vi "Open Sensors and Actuators.vi"   [LabVIEW 2014]
uses:
  <vilib>/Rock Robotics/SystemInterfaces/DIO/FPGA_DIOPWMChannel.ctl
  <vilib>/Rock Robotics/WPI/Joystick/WPI_JoystickDeviceEnum.ctl
  <vilib>/Rock Robotics/SystemInterfaces/DIO/FPGA_DIOChannel.ctl
  <vilib>/Rock Robotics/WPI/Solenoid/WPI_SolenoidChannel.ctl
  <vilib>/Rock Robotics/SystemInterfaces/AI/FPGA_AIChannel.ctl
  <vilib>/Rock Robotics/WPI/MotorControl/WPI_MotorControlOpen Talon.vi
  <vilib>/Rock Robotics/WPI/Counter/WPI_CounterDigitalInputToDigitalSource.vi
  <vilib>/Rock Robotics/WPI/Solenoid/WPI_SolenoidOpenSingle.vi
  <vilib>/Rock Robotics/WPI/Counter/WPI_CounterOpen UpDown Mode.vi
  <vilib>/Rock Robotics/WPI/Switch/WPI_SwitchOpenLimit.vi
  <vilib>/Rock Robotics/WPI/Ultrasonic/WPI_SonarMB1010AnalogOpen.vi
  Global RefNums.vi
  <vilib>/Rock Robotics/WPI/Compressor/WPI_CompressorGetSetRefNum.vi
  <vilib>/Rock Robotics/WPI/Ultrasonic/WPI_SonarMB1010AnalogRefNum Registry Set.vi
  _Dependencies/NavX/navX-MXP IMU.lvlib
types:
  T1 = typedef "WPI_SolenoidChannel.ctl" = enum8{"Solenoid 0", "Solenoid 1", "Solenoid 2", "Solenoid 3", "Solenoid 4", "Solenoid 5", "Solenoid 6", "Solenoid 7", "Invalid"}
  T2 = typedef "FPGA_AIChannel.ctl" = enum8{"AI 0", "AI 1", "AI 2", "AI 3", "AI MXP 0", "AI MXP 1", "AI MXP 2", "AI MXP 3", "Invalid"}
  T3 = typedef "FPGA_DIOChannel.ctl" = enum8{"DIO 0", "DIO 1", "DIO 2", "DIO 3", "DIO 4", "DIO 5", "DIO 6", "DIO 7", "DIO 8", "DIO 9", "DIO MXP 0", "DIO MXP 1", "DIO MXP 2", "DIO MXP 3", "DIO MXP 4", "DIO MXP 5", "DIO MXP 6", "DIO MXP 7", "DIO MXP 8", "DIO MXP 9", "DIO MXP 10", "DIO MXP 11", "DIO MXP 12", "DIO MXP 13", "DIO MXP 14", "DIO MXP 15", "Invalid"}
  T4 = typedef "FPGA_DIOPWMChannel.ctl" = enum8{"PWM 0", "PWM 1", "PWM 2", "PWM 3", "PWM 4", "PWM 5", "PWM 6", "PWM 7", "PWM 8", "PWM 9", "PWM MXP 0", "PWM MXP 1", "PWM MXP 2", "PWM MXP 3", "PWM MXP 4", "PWM MXP 5", "PWM MXP 6", "PWM MXP 7", "PWM MXP 8", "PWM MXP 9", "Invalid"}
  T5 = enum16{"Rising Edge", "Falling Edge", "Raising & Falling Edge", "Disabled"}
  T6 = typedef "WPI_JoystickDeviceEnum.ctl" = enum16{"USB 0", "USB 1", "USB 2", "USB 3", "USB 4", "USB 5"}
  T7 = typedef "WPI_MotorControlDeviceRef.ctl" = cluster{"DeviceStatus":errorcluster, "Type":T8, "PWM":cluster{"Controller":T9, "PWM Channel":T4, "DeadBand":T10}, "CAN":cluster{"Device Number":u8, "Control Mode":T11, "Semaphore":T12, "Max Vout":dbl, "TalonSRX Control Mode":T13}, "Invert":bool, "TransformRef":T14, "InvTransformRef":T14}
  T8 = typedef "WPI_MotorControlType.ctl" = enum16{"PWM", "CAN", "CANTalonSRX"}
  T9 = typedef "FPGA_TypedefDigitalModule.ctl" = enum16{"Controller 1"}
  T10 = typedef "WPI_PWMDeadband.ctl" = cluster{"Name":string, "maxPositivePwm":i32, "minPositivePwm":i32, "centerPwm":i32, "maxNegativePwm":i32, "minNegativePwm":i32, "angularRange":u16}
  T11 = typedef "WPI_CANJaguar_ControlMode.ctl" = enum8{"Percent VBus", "Current", "Speed", "Position", "Voltage"}
  T12 = typedef "Semaphore RefNum" = refnum<k1>
  T13 = typedef "WPI_CANTalonSRX_APIControlMode.ctl" = enum8{"Percent VBus", "Speed", "Position", "Slave", "Unchanged / Invalid"}
  T14 = typedef "WPI_PWMTransform_ConPane.ctl" = refnum<vi>
  T15 = typedef "WPI_DigitalInputDevRef.ctl" = cluster{"DevStatus":errorcluster, "DIO Channel":T3, "Controller":T9}
  T16 = typedef "FPGA_CounterEncoderSourceConvertionLVSourceType.ctl" = cluster{"DevStatus":errorcluster, "AnalogTriggerMode?":bool, "DigitalMode":cluster{"Controller":T9, "DIO Channel":T17}, "AnalogTriggerMode":cluster{"AnalogTriggerIndex":T18, "OutputType":T19}}
  T17 = typedef "FPGA_DIODigitalSourceChannel.ctl" = enum8{"DIO 0", "DIO 1", "DIO 2", "DIO 3", "DIO 4", "DIO 5", "DIO 6", "DIO 7", "DIO 8", "DIO 9", "DIO MXP 0", "DIO MXP 1", "DIO MXP 2", "DIO MXP 3", "DIO MXP 4", "DIO MXP 5", "DIO MXP 6", "DIO MXP 7", "DIO MXP 8", "DIO MXP 9", "DIO MXP 10", "DIO MXP 11", "DIO MXP 12", "DIO MXP 13", "DIO MXP 14", "DIO MXP 15", "Disabled"}
  T18 = typedef "FPGA_AnalogTriggerIndex.ctl" = enum8{"Trig 0", "Trig 1", "Trig 2", "Trig 3", "Trig 4", "Trig 5", "Trig 6", "Trig 7", "Invalid"}
  T19 = typedef "FPGA_AnalogTriggerOutType.ctl" = enum16{"InWindow", "TriggerState", "Rising", "Falling"}
  T20 = typedef "WPI_EncoderDevRef.ctl" = cluster{"DevStatus":errorcluster, "EncoderIndex":T21, "CounterIndex":T22, "DistancePerCount":dbl, "Decoding Type":T23}
  T21 = typedef "FPGA_EncoderIdx.ctl" = enum8{"Enc 0", "Enc 1", "Enc 2", "Enc 3", "Enc 4", "Enc 5", "Enc 6", "Enc 7", "Invalid"}
  T22 = typedef "FPGA_CounterCtrSystemIndex.ctl" = enum8{"Ctr 0", "Ctr 1", "Ctr 2", "Ctr 3", "Ctr 4", "Ctr 5", "Ctr 6", "Ctr 7", "Invalid"}
  T23 = typedef "WPI_EncoderType.ctl" = enum16{"1x", "2x", "4x"}
  T24 = typedef "navX-MXP IMU.lvlib/navX Device TypeDef.ctl" = cluster{"navX Interface Protocol":T25, "navX Interface Protocol TypeDefs":cluster{"SPIDevRef":T26, "I2CDevRef":T28}, "navX System Information":cluster{"Board Information":T30, "Status":T31, "Offsets":T35}, "navX Common Information":cluster{"Update Rate (4Hz-60Hz)":T36, "refnum name":string, "error":errorcluster}}
  T25 = typedef "navX-MXP IMU.lvlib/navX Interface Protocol.ctl" = enum16{"SPI", "I2C"}
  T26 = typedef "WPI_SPIDevRef.ctl" = cluster{"DevStatus":errorcluster, "Handle":i32, "Controller":T9, "SPI Bus":T27}
  T27 = typedef "spi_bus.ctl" = enum16{"SPI On-Board, CS0", "SPI On-Board, CS1", "SPI On-Board, CS2", "SPI On-Board, CS3", "SPI MXP", "Invalid"}
  T28 = typedef "WPI_I2CDevRef.ctl" = cluster{"DevStatus":errorcluster, "Controller":T9, "Device Address":u8, "Handle":i32, "I2C Bus":T29}
  T29 = typedef "i2c_bus.ctl" = enum16{"I2C On-Board", "I2C MXP", "Invalid"}
  T30 = typedef "navX-MXP IMU.lvlib/navX Board Information.ctl" = cluster{"WhoAmI (50 | 0x32)":u8, "Board Revision":u8, "Firmware Major Version":u8, "Firmware Minor Version":u8}
  T31 = typedef "navX-MXP IMU.lvlib/navX Status Data.ctl" = cluster{"Update Rate Hz":u8, "Accelerometer Full-Scale Range":u8, "Gyro Full-Scale Range":u16, "NAVX_OP_STATUS":T32, "NAVX_CAL_STATUS":T33, "NAVX_SELFTEST_STATUS":u8, "NAVX_SENSOR_STATUS":T34}
  T32 = typedef "navX-MXP IMU.lvlib/navX NAVX_OP_STATUS.ctl" = u8
  T33 = typedef "navX-MXP IMU.lvlib/navX NAVX_CAL_STATUS.ctl" = u8
  T34 = typedef "navX-MXP IMU.lvlib/navX NAVX_SENSOR_STATUS.ctl" = cluster{"MOVING":bool, "YAW_STABLE":bool, "MAG_DISTURBANCE":bool, "ALTITUDE_VALID":bool, "SEALEVEL_PRESS_SET":bool, "FUSED_HEADING_VALID":bool}
  T35 = typedef "navX-MXP IMU.lvlib/navX Offsets Data.ctl" = cluster{"Yaw":dbl, "Quat W":dbl, "Quat X":dbl, "Quat Y":dbl, "Quat Z":dbl}
  T36 = typedef "navX-MXP IMU.lvlib/navX Update Rate.ctl" = u8
  T37 = typedef "WPI_JoystickDevRef.ctl" = cluster{"Device":T6}
  T38 = typedef "WPI_SolenoidDevRef.ctl" = cluster{"DevStatus":errorcluster, "Pneumatics Control Module":u8, "Forward Solenoid Channel":T1, "Reverse Solenoid Channel":T1}
  T39 = typedef "WPI_AnalogChannelDevRef.ctl" = cluster{"DevStatus":errorcluster, "Controller":T40, "Analog Channel":T2}
  T40 = typedef "FPGA_TypedefAnalogModule.ctl" = enum16{"Controller 1"}
  T41 = typedef "WPI_CounterDevRef.ctl" = cluster{"DevStatus":errorcluster, "CntIndex":T22}
  T42 = typedef "WPI_CompressorDevRef.ctl" = cluster{"DevStatus":errorcluster, "Pneumatics Control Module":u8}
  T43 = typedef "WPI_SwitchDevRef.ctl" = cluster{"DevStatus":errorcluster, "DIO Channel":T3, "Controller":T9, "CntIndex":T22, "Normally Closed":bool}
  T44 = typedef "WPI_SonarMB1010AnalogDeviceRef.ctl" = cluster{"AIDeviceRef":T39, "Scaling factor (V/in)":dbl, "Average Bits":u8}
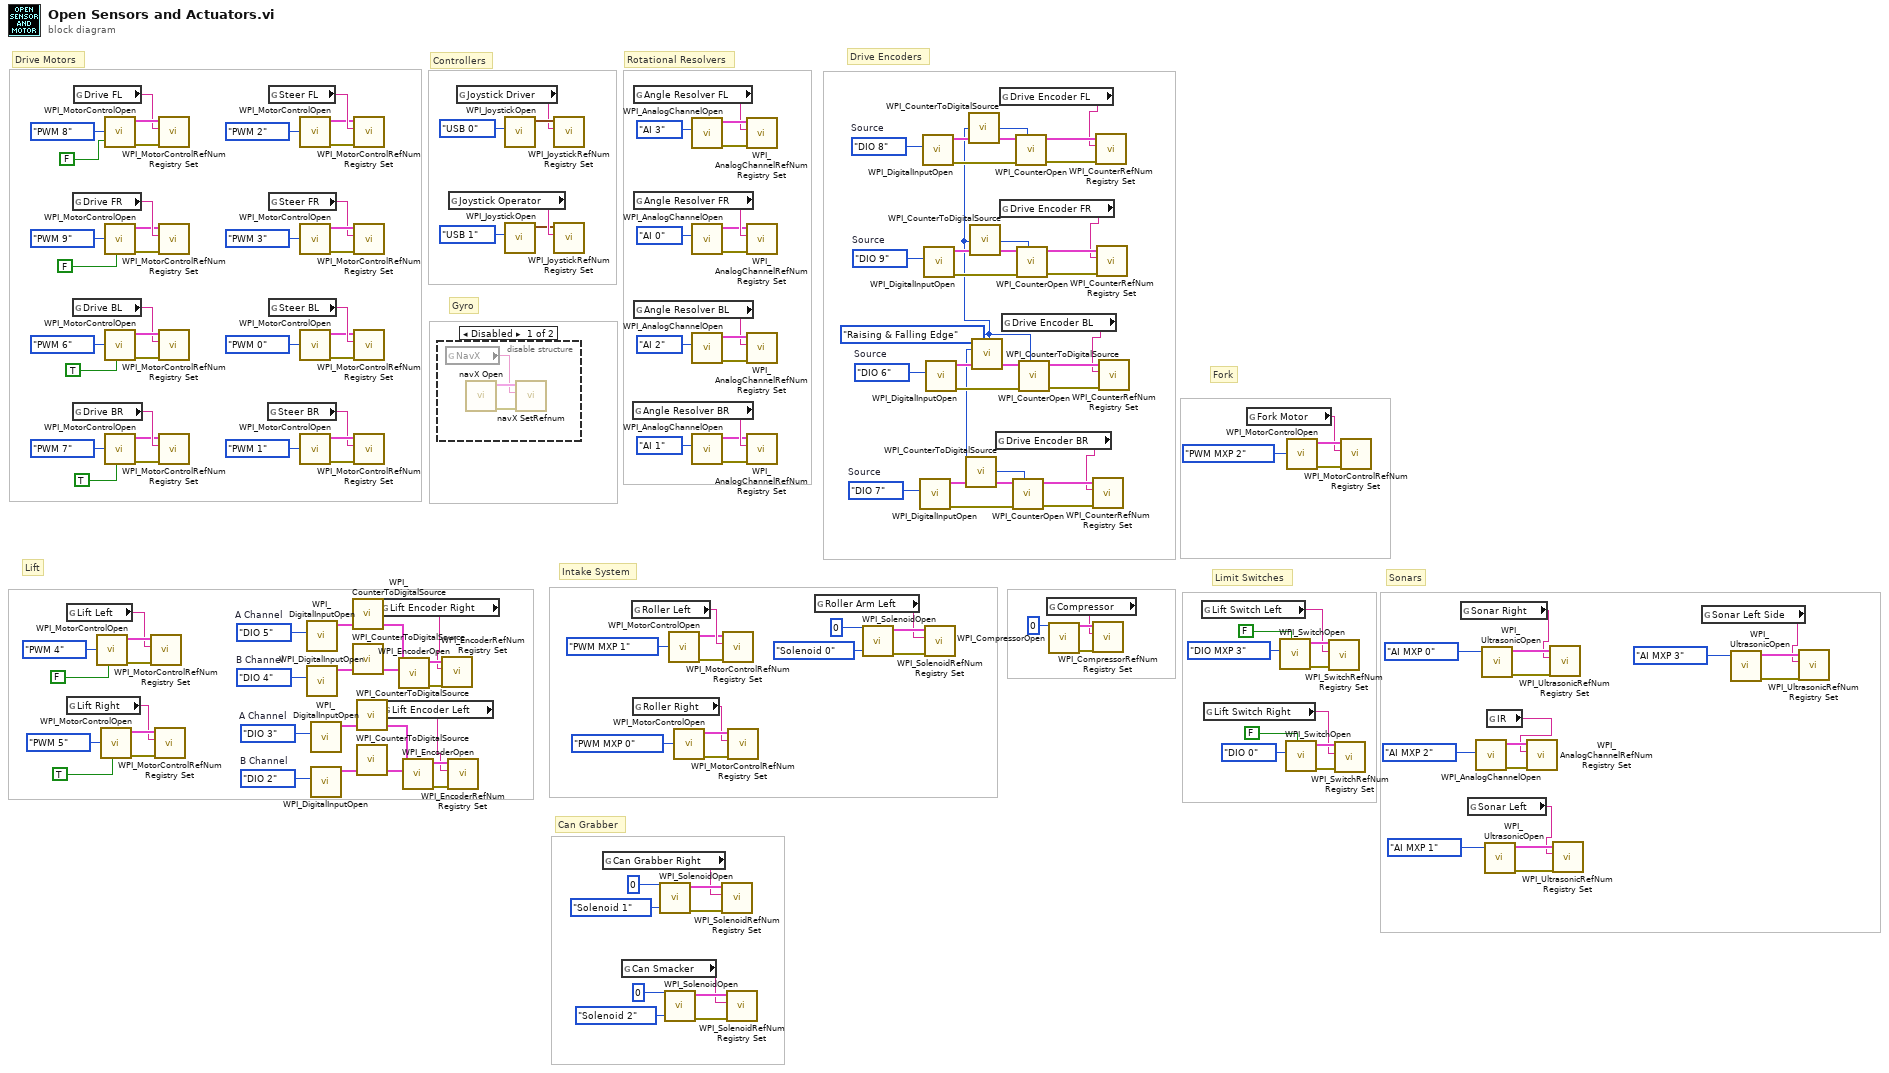
[diagram p0: block diagram]
diagram:
  w57 = T5."Raising & Falling Edge" ("UpEdge")
  w67 = FPGA_DIOChannel."DIO 7"  # Source
  w74 = FPGA_DIOChannel."DIO 6"  # Source
  w81 = FPGA_DIOChannel."DIO 9"  # Source
  w109 = FPGA_DIOChannel."DIO 2"  # B Channel
  w108 = FPGA_DIOChannel."DIO 3"  # A Channel
  w115 = FPGA_DIOChannel."DIO 4"  # B Channel
  w114 = FPGA_DIOChannel."DIO 5"  # A Channel
  w133 = FPGA_DIOChannel."DIO 8"  # Source
  # "Can Grabber"
  # "Sonars"
  # "Limit Switches"
  # "Fork"
  # "Intake System"
  # "Gyro"
  # "Drive Encoders"
  # "Lift"
  # "Drive Motors"
  # "Controllers"
  # "Rotational Resolvers"
  n1 = global read "Global RefNums.vi" "Lift Left"() -> (w125:string)
  n2 = global read "Global RefNums.vi" "Lift Right"() -> (w121:string)
  n3 = global read "Global RefNums.vi" "Drive FR"() -> (w166:string)
  n4 = global read "Global RefNums.vi" "Drive BL"() -> (w161:string)
  n5 = global read "Global RefNums.vi" "Drive BR"() -> (w158:string)
  n6 = global read "Global RefNums.vi" "Drive FL"() -> (w169:string)
  n7 = call-poly <vilib>:"WPI_MotorControlOpen.vi"("Invert"=FALSE, "PWM Channel"=FPGA_DIOPWMChannel."PWM 4") -> ("error out"=w126:errorcluster, "MotorControlDeviceRef"=w127:T7)  [unwired: 8 in]
  n8 = call-poly <vilib>:"WPI_MotorControlOpen.vi"("Invert"=TRUE, "PWM Channel"=FPGA_DIOPWMChannel."PWM 5") -> ("error out"=w122:errorcluster, "MotorControlDeviceRef"=w123:T7)  [unwired: 8 in]
  n9 = call-poly <vilib>:"WPI_MotorControlOpen.vi"("Invert"=FALSE, "PWM Channel"=FPGA_DIOPWMChannel."PWM 8") -> ("error out"=w170:errorcluster, "MotorControlDeviceRef"=w171:T7)  [unwired: 8 in]
  n10 = call-poly <vilib>:"WPI_MotorControlOpen.vi"("Invert"=FALSE, "PWM Channel"=FPGA_DIOPWMChannel."PWM 9") -> ("error out"=w165:errorcluster, "MotorControlDeviceRef"=w164:T7)  [unwired: 8 in]
  n11 = call-poly <vilib>:"WPI_MotorControlOpen.vi"("Invert"=TRUE, "PWM Channel"=FPGA_DIOPWMChannel."PWM 6") -> ("error out"=w162:errorcluster, "MotorControlDeviceRef"=w163:T7)  [unwired: 8 in]
  n12 = call-poly <vilib>:"WPI_MotorControlOpen.vi"("Invert"=TRUE, "PWM Channel"=FPGA_DIOPWMChannel."PWM 7") -> ("error out"=w157:errorcluster, "MotorControlDeviceRef"=w156:T7)  [unwired: 8 in]
  n13 = call <vilib>:"WPI_MotorControlRefNum Registry Set.vi"("error in (no error)"=w126, "refnum name"=w125, "MotorControlDevRef"=w127) -> ()  [unwired: 7 in, 2 out]
  n14 = call <vilib>:"WPI_MotorControlRefNum Registry Set.vi"("error in (no error)"=w122, "refnum name"=w121, "MotorControlDevRef"=w123) -> ()  [unwired: 7 in, 2 out]
  n15 = call <vilib>:"WPI_MotorControlRefNum Registry Set.vi"("error in (no error)"=w170, "refnum name"=w169, "MotorControlDevRef"=w171) -> ()  [unwired: 7 in, 2 out]
  n16 = call <vilib>:"WPI_MotorControlRefNum Registry Set.vi"("error in (no error)"=w165, "refnum name"=w166, "MotorControlDevRef"=w164) -> ()  [unwired: 7 in, 2 out]
  n17 = call <vilib>:"WPI_MotorControlRefNum Registry Set.vi"("error in (no error)"=w162, "refnum name"=w161, "MotorControlDevRef"=w163) -> ()  [unwired: 7 in, 2 out]
  n18 = call <vilib>:"WPI_MotorControlRefNum Registry Set.vi"("error in (no error)"=w157, "refnum name"=w158, "MotorControlDevRef"=w156) -> ()  [unwired: 7 in, 2 out]
  n19 = global read "Global RefNums.vi" "Steer BR"() -> (w153:string)
  n20 = global read "Global RefNums.vi" "Steer FL"() -> (w142:string)
  n21 = global read "Global RefNums.vi" "Steer FR"() -> (w145:string)
  n22 = global read "Global RefNums.vi" "Steer BL"() -> (w150:string)
  n23 = call-poly <vilib>:"WPI_MotorControlOpen.vi"("PWM Channel"=FPGA_DIOPWMChannel."PWM 2") -> ("error out"=w141:errorcluster, "MotorControlDeviceRef"=w140:T7)  [unwired: 9 in]
  n24 = call-poly <vilib>:"WPI_MotorControlOpen.vi"("PWM Channel"=FPGA_DIOPWMChannel."PWM 3") -> ("error out"=w146:errorcluster, "MotorControlDeviceRef"=w147:T7)  [unwired: 9 in]
  n25 = call-poly <vilib>:"WPI_MotorControlOpen.vi"("PWM Channel"=FPGA_DIOPWMChannel."PWM 0") -> ("error out"=w149:errorcluster, "MotorControlDeviceRef"=w148:T7)  [unwired: 9 in]
  n26 = call-poly <vilib>:"WPI_MotorControlOpen.vi"("PWM Channel"=FPGA_DIOPWMChannel."PWM 1") -> ("error out"=w154:errorcluster, "MotorControlDeviceRef"=w155:T7)  [unwired: 9 in]
  n27 = call <vilib>:"WPI_DigitalInputOpen.vi"("DIO Channel"=w114) -> ("DigitalInputDevRef"=w111:T15)  [unwired: 2 in, 8 out]
  n28 = call <vilib>:"WPI_DigitalInputOpen.vi"("DIO Channel"=w115) -> ("DigitalInputDevRef"=w112:T15)  [unwired: 2 in, 8 out]
  n29 = call <vilib>:"WPI_DigitalInputOpen.vi"("DIO Channel"=w108) -> ("DigitalInputDevRef"=w105:T15)  [unwired: 2 in, 8 out]
  n30 = call <vilib>:"WPI_DigitalInputOpen.vi"("DIO Channel"=w109) -> ("DigitalInputDevRef"=w106:T15)  [unwired: 2 in, 8 out]
  n31 = call-poly <vilib>:"WPI_CounterToDigitalSource.vi"("DigitalInputDevRef"=w111) -> ("Digital Source"=w110:T16)  [unwired: 6 out]
  n32 = call-poly <vilib>:"WPI_CounterToDigitalSource.vi"("DigitalInputDevRef"=w112) -> ("Digital Source"=w113:T16)  [unwired: 6 out]
  n33 = call <vilib>:"WPI_MotorControlRefNum Registry Set.vi"("error in (no error)"=w141, "refnum name"=w142, "MotorControlDevRef"=w140) -> ()  [unwired: 7 in, 2 out]
  n34 = call <vilib>:"WPI_MotorControlRefNum Registry Set.vi"("error in (no error)"=w146, "refnum name"=w145, "MotorControlDevRef"=w147) -> ()  [unwired: 7 in, 2 out]
  n35 = call <vilib>:"WPI_MotorControlRefNum Registry Set.vi"("error in (no error)"=w149, "refnum name"=w150, "MotorControlDevRef"=w148) -> ()  [unwired: 7 in, 2 out]
  n36 = call <vilib>:"WPI_MotorControlRefNum Registry Set.vi"("error in (no error)"=w154, "refnum name"=w153, "MotorControlDevRef"=w155) -> ()  [unwired: 7 in, 2 out]
  n37 = call-poly <vilib>:"WPI_CounterToDigitalSource.vi"("DigitalInputDevRef"=w105) -> ("Digital Source"=w104:T16)  [unwired: 6 out]
  n38 = call-poly <vilib>:"WPI_CounterToDigitalSource.vi"("DigitalInputDevRef"=w106) -> ("Digital Source"=w107:T16)  [unwired: 6 out]
  n39 = global read "Global RefNums.vi" "Lift Encoder Right"() -> (w98:string)
  n40 = global read "Global RefNums.vi" "Lift Encoder Left"() -> (w99:string)
  n41 = call <vilib>:"WPI_EncoderOpen.vi"("BSource"=w113, "ASource"=w110) -> ("error out"=w103:errorcluster, "EncoderDevRef"=w102:T20)  [unwired: 6 in, 2 out]
  n42 = call <vilib>:"WPI_EncoderOpen.vi"("BSource"=w107, "ASource"=w104) -> ("error out"=w101:errorcluster, "EncoderDevRef"=w100:T20)  [unwired: 6 in, 2 out]
  n43 = disable-structure shown="Disabled" {
    frame Disabled {
      n44 = global read "Global RefNums.vi" "NavX"() -> (w173:string)
      n45 = call "navX Open.vi"() -> ("error out"=w175:errorcluster, "navX Device TypeDef"=w174:T24)  [unwired: 9 in, 1 out]
      n46 = call "navX SetRefnum.vi"("error in (no error)"=w175, "refnum name"=w173, "navX Device TypeDef"=w174) -> ()  [unwired: 7 in, 2 out]
    }
    frame Enabled {
    }
  }
  n47 = call <vilib>:"WPI_EncoderRefNum Registry Set.vi"("error in (no error)"=w103, "refnum name"=w98, "EncoderDevRef"=w102) -> ()  [unwired: 7 in, 2 out]
  n48 = call <vilib>:"WPI_EncoderRefNum Registry Set.vi"("error in (no error)"=w101, "refnum name"=w99, "EncoderDevRef"=w100) -> ()  [unwired: 7 in, 2 out]
  n49 = global read "Global RefNums.vi" "Joystick Operator"() -> (w138:string)
  n50 = global read "Global RefNums.vi" "Joystick Driver"() -> (w139:string)
  n51 = call <vilib>:"WPI_JoystickOpen.vi"("JoystickDevice"=WPI_JoystickDeviceEnum."USB 0") -> ("JoystickDevRef"=w172:T37)  [unwired: 10 in]
  n52 = call <vilib>:"WPI_JoystickOpen.vi"("JoystickDevice"=WPI_JoystickDeviceEnum."USB 1") -> ("JoystickDevRef"=w137:T37)  [unwired: 10 in]
  n53 = call <vilib>:"WPI_JoystickRefNum Registry Set.vi"("refnum name"=w139, "JoystickDevRef"=w172) -> ()  [unwired: 8 in, 2 out]
  n54 = call <vilib>:"WPI_JoystickRefNum Registry Set.vi"("refnum name"=w138, "JoystickDevRef"=w137) -> ()  [unwired: 8 in, 2 out]
  n55 = global read "Global RefNums.vi" "Can Grabber Right"() -> (w6:string)
  n56 = global read "Global RefNums.vi" "Can Smacker"() -> (w1:string)
  n57 = global read "Global RefNums.vi" "Roller Left"() -> (w94:string)
  n58 = global read "Global RefNums.vi" "Angle Resolver BR"() -> (w25:string)
  n59 = global read "Global RefNums.vi" "Roller Right"() -> (w89:string)
  n60 = global read "Global RefNums.vi" "Angle Resolver FL"() -> (w36:string)
  n61 = global read "Global RefNums.vi" "Angle Resolver FR"() -> (w33:string)
  n62 = global read "Global RefNums.vi" "Angle Resolver BL"() -> (w28:string)
  n63 = call-poly <vilib>:"WPI_SolenoidOpen.vi"("Solenoid Channel"=WPI_SolenoidChannel."Solenoid 1", "Pneumatics Control Module (0)"=u8 0) -> ("error out"=w9:errorcluster, "SolenoidDevRef"=w10:T38)  [unwired: 8 in]
  n64 = call-poly <vilib>:"WPI_SolenoidOpen.vi"("Solenoid Channel"=WPI_SolenoidChannel."Solenoid 2", "Pneumatics Control Module (0)"=u8 0) -> ("error out"=w4:errorcluster, "SolenoidDevRef"=w5:T38)  [unwired: 8 in]
  n65 = call-poly <vilib>:"WPI_MotorControlOpen.vi"("PWM Channel"=FPGA_DIOPWMChannel."PWM MXP 1") -> ("error out"=w93:errorcluster, "MotorControlDeviceRef"=w92:T7)  [unwired: 9 in]
  n66 = call-poly <vilib>:"WPI_MotorControlOpen.vi"("PWM Channel"=FPGA_DIOPWMChannel."PWM MXP 0") -> ("error out"=w90:errorcluster, "MotorControlDeviceRef"=w91:T7)  [unwired: 9 in]
  n67 = call <vilib>:"WPI_AnalogChannelOpen.vi"("Analog Channel"=FPGA_AIChannel."AI 3") -> ("error out"=w38:errorcluster, "AIDeviceRef"=w37:T39)  [unwired: 9 in]
  n68 = call <vilib>:"WPI_AnalogChannelOpen.vi"("Analog Channel"=FPGA_AIChannel."AI 0") -> ("error out"=w31:errorcluster, "AIDeviceRef"=w32:T39)  [unwired: 9 in]
  n69 = call <vilib>:"WPI_AnalogChannelOpen.vi"("Analog Channel"=FPGA_AIChannel."AI 2") -> ("error out"=w30:errorcluster, "AIDeviceRef"=w29:T39)  [unwired: 9 in]
  n70 = call <vilib>:"WPI_AnalogChannelOpen.vi"("Analog Channel"=FPGA_AIChannel."AI 1") -> ("error out"=w23:errorcluster, "AIDeviceRef"=w24:T39)  [unwired: 9 in]
  n71 = call <vilib>:"WPI_SolenoidRefNum Registry Set.vi"("error in (no error)"=w9, "refnum name"=w6, "SolenoidDevRef"=w10) -> ()  [unwired: 7 in, 2 out]
  n72 = call <vilib>:"WPI_MotorControlRefNum Registry Set.vi"("error in (no error)"=w93, "refnum name"=w94, "MotorControlDevRef"=w92) -> ()  [unwired: 7 in, 2 out]
  n73 = call <vilib>:"WPI_SolenoidRefNum Registry Set.vi"("error in (no error)"=w4, "refnum name"=w1, "SolenoidDevRef"=w5) -> ()  [unwired: 7 in, 2 out]
  n74 = call <vilib>:"WPI_MotorControlRefNum Registry Set.vi"("error in (no error)"=w90, "refnum name"=w89, "MotorControlDevRef"=w91) -> ()  [unwired: 7 in, 2 out]
  n75 = call <vilib>:"WPI_AnalogChannelRefNum Registry Set.vi"("error in (no error)"=w38, "refnum name"=w36, "AIDeviceRef"=w37) -> ()  [unwired: 7 in, 2 out]
  n76 = call <vilib>:"WPI_AnalogChannelRefNum Registry Set.vi"("error in (no error)"=w31, "refnum name"=w33, "AIDeviceRef"=w32) -> ()  [unwired: 7 in, 2 out]
  n77 = call <vilib>:"WPI_AnalogChannelRefNum Registry Set.vi"("error in (no error)"=w30, "refnum name"=w28, "AIDeviceRef"=w29) -> ()  [unwired: 7 in, 2 out]
  n78 = call <vilib>:"WPI_AnalogChannelRefNum Registry Set.vi"("error in (no error)"=w23, "refnum name"=w25, "AIDeviceRef"=w24) -> ()  [unwired: 7 in, 2 out]
  n79 = global read "Global RefNums.vi" "Roller Arm Left"() -> (w83:string)
  n80 = call-poly <vilib>:"WPI_SolenoidOpen.vi"("Solenoid Channel"=WPI_SolenoidChannel."Solenoid 0", "Pneumatics Control Module (0)"=u8 0) -> ("error out"=w86:errorcluster, "SolenoidDevRef"=w87:T38)  [unwired: 8 in]
  n81 = call <vilib>:"WPI_DigitalInputOpen.vi"("DIO Channel"=w67) -> ("error out"=w63:errorcluster, "DigitalInputDevRef"=w66:T15)  [unwired: 2 in, 7 out]
  n82 = call <vilib>:"WPI_DigitalInputOpen.vi"("DIO Channel"=w133) -> ("error out"=w129:errorcluster, "DigitalInputDevRef"=w132:T15)  [unwired: 2 in, 7 out]
  n83 = call <vilib>:"WPI_DigitalInputOpen.vi"("DIO Channel"=w81) -> ("error out"=w77:errorcluster, "DigitalInputDevRef"=w80:T15)  [unwired: 2 in, 7 out]
  n84 = call <vilib>:"WPI_SolenoidRefNum Registry Set.vi"("error in (no error)"=w86, "refnum name"=w83, "SolenoidDevRef"=w87) -> ()  [unwired: 7 in, 2 out]
  n85 = call <vilib>:"WPI_DigitalInputOpen.vi"("DIO Channel"=w74) -> ("error out"=w70:errorcluster, "DigitalInputDevRef"=w73:T15)  [unwired: 2 in, 7 out]
  n86 = call-poly <vilib>:"WPI_CounterToDigitalSource.vi"("DigitalInputDevRef"=w66) -> ("Digital Source"=w68:T16)  [unwired: 6 out]
  n87 = call-poly <vilib>:"WPI_CounterToDigitalSource.vi"("DigitalInputDevRef"=w132) -> ("Digital Source"=w134:T16)  [unwired: 6 out]
  n88 = call-poly <vilib>:"WPI_CounterToDigitalSource.vi"("DigitalInputDevRef"=w80) -> ("Digital Source"=w82:T16)  [unwired: 6 out]
  n89 = call-poly <vilib>:"WPI_CounterToDigitalSource.vi"("DigitalInputDevRef"=w73) -> ("Digital Source"=w75:T16)  [unwired: 6 out]
  n90 = global read "Global RefNums.vi" "Drive Encoder BR"() -> (w62:string)
  n91 = global read "Global RefNums.vi" "Drive Encoder FL"() -> (w128:string)
  n92 = global read "Global RefNums.vi" "Drive Encoder FR"() -> (w76:string)
  n93 = global read "Global RefNums.vi" "Drive Encoder BL"() -> (w69:string)
  n94 = call-poly <vilib>:"WPI_CounterOpen.vi"("UpEdge"=w57, "error in (no error)"=w63, "Up Source"=w68) -> ("error out"=w64:errorcluster, "CounterDevRef"=w65:T41)  [unwired: 4 in, 3 out]
  n95 = call-poly <vilib>:"WPI_CounterOpen.vi"("UpEdge"=w57, "error in (no error)"=w129, "Up Source"=w134) -> ("error out"=w130:errorcluster, "CounterDevRef"=w131:T41)  [unwired: 4 in, 3 out]
  n96 = call-poly <vilib>:"WPI_CounterOpen.vi"("UpEdge"=w57, "error in (no error)"=w77, "Up Source"=w82) -> ("error out"=w78:errorcluster, "CounterDevRef"=w79:T41)  [unwired: 4 in, 3 out]
  n97 = call-poly <vilib>:"WPI_CounterOpen.vi"("UpEdge"=w57, "error in (no error)"=w70, "Up Source"=w75) -> ("error out"=w71:errorcluster, "CounterDevRef"=w72:T41)  [unwired: 4 in, 3 out]
  n98 = global read "Global RefNums.vi" "Compressor"() -> (w58:string)
  n99 = call <vilib>:"WPI_CompressorOpen.vi"("Pneumatics Control Module (0)"=u8 0) -> ("CompressorDevRef"=w61:T42, "error out"=w60:errorcluster)  [unwired: 13 in]
  n100 = call <vilib>:"WPI_CounterRefNum Registry Set.vi"("error in (no error)"=w64, "refnum name"=w62, "CounterDevRef"=w65) -> ()  [unwired: 7 in, 2 out]
  n101 = call <vilib>:"WPI_CompressorRefNum Registry Set.vi"("error in (no error)"=w60, "refnum name"=w58, "CompressorDevRef"=w61) -> ()  [unwired: 7 in, 2 out]
  n102 = call <vilib>:"WPI_CounterRefNum Registry Set.vi"("error in (no error)"=w130, "refnum name"=w128, "CounterDevRef"=w131) -> ()  [unwired: 7 in, 2 out]
  n103 = call <vilib>:"WPI_CounterRefNum Registry Set.vi"("error in (no error)"=w78, "refnum name"=w76, "CounterDevRef"=w79) -> ()  [unwired: 7 in, 2 out]
  n104 = call <vilib>:"WPI_CounterRefNum Registry Set.vi"("error in (no error)"=w71, "refnum name"=w69, "CounterDevRef"=w72) -> ()  [unwired: 7 in, 2 out]
  n105 = global read "Global RefNums.vi" "Lift Switch Left"() -> (w48:string)
  n106 = global read "Global RefNums.vi" "Lift Switch Right"() -> (w43:string)
  n107 = global read "Global RefNums.vi" "Fork Motor"() -> (w50:string)
  n108 = call-poly <vilib>:"WPI_SwitchOpen.vi"("Normally Closed"=FALSE, "DIO Channel"=FPGA_DIOChannel."DIO MXP 3") -> ("error out"=w56:errorcluster, "SwitchDevRef"=w55:T43)  [unwired: 8 in]
  n109 = call-poly <vilib>:"WPI_SwitchOpen.vi"("Normally Closed"=FALSE, "DIO Channel"=FPGA_DIOChannel."DIO 0") -> ("error out"=w47:errorcluster, "SwitchDevRef"=w46:T43)  [unwired: 8 in]
  n110 = call-poly <vilib>:"WPI_MotorControlOpen.vi"("PWM Channel"=FPGA_DIOPWMChannel."PWM MXP 2") -> ("error out"=w51:errorcluster, "MotorControlDeviceRef"=w52:T7)  [unwired: 9 in]
  n111 = call <vilib>:"WPI_SwitchRefNum Registry Set.vi"("error in (no error)"=w56, "refnum name"=w48, "SwitchDevRef"=w55) -> ()  [unwired: 7 in, 2 out]
  n112 = call <vilib>:"WPI_SwitchRefNum Registry Set.vi"("error in (no error)"=w47, "refnum name"=w43, "SwitchDevRef"=w46) -> ()  [unwired: 7 in, 2 out]
  n113 = call <vilib>:"WPI_MotorControlRefNum Registry Set.vi"("error in (no error)"=w51, "refnum name"=w50, "MotorControlDevRef"=w52) -> ()  [unwired: 7 in, 2 out]
  n114 = global read "Global RefNums.vi" "Sonar Right"() -> (w40:string)
  n115 = global read "Global RefNums.vi" "Sonar Left"() -> (w12:string)
  n116 = call <vilib>:"WPI_AnalogChannelOpen.vi"("Analog Channel"=FPGA_AIChannel."AI MXP 2") -> ("error out"=w22:errorcluster, "AIDeviceRef"=w21:T39)  [unwired: 9 in]
  n117 = call-poly <vilib>:"WPI_UltrasonicOpen.vi"("Analog Channel"=FPGA_AIChannel."AI MXP 0") -> ("error out"=w42:errorcluster, "SonarMB1010AnalogDevRef"=w41:T44)  [unwired: 9 in]
  n118 = call-poly <vilib>:"WPI_UltrasonicOpen.vi"("Analog Channel"=FPGA_AIChannel."AI MXP 1") -> ("error out"=w14:errorcluster, "SonarMB1010AnalogDevRef"=w13:T44)  [unwired: 9 in]
  n119 = global read "Global RefNums.vi" "IR"() -> (w20:string)
  n120 = call <vilib>:"WPI_AnalogChannelRefNum Registry Set.vi"("error in (no error)"=w22, "refnum name"=w20, "AIDeviceRef"=w21) -> ()  [unwired: 7 in, 2 out]
  n121 = call-poly <vilib>:"WPI_UltrasonicRefNum Registry Set.vi"("error in (no error)"=w42, "refnum name"=w40, "SonarMB1010AnalogDevRef"=w41) -> ()  [unwired: 7 in, 2 out]
  n122 = call-poly <vilib>:"WPI_UltrasonicRefNum Registry Set.vi"("error in (no error)"=w14, "refnum name"=w12, "SonarMB1010AnalogDevRef"=w13) -> ()  [unwired: 7 in, 2 out]
  n123 = global read "Global RefNums.vi" "Sonar Left Side"() -> (w16:string)
  n124 = call-poly <vilib>:"WPI_UltrasonicOpen.vi"("Analog Channel"=FPGA_AIChannel."AI MXP 3") -> ("error out"=w18:errorcluster, "SonarMB1010AnalogDevRef"=w17:T44)  [unwired: 9 in]
  n125 = call-poly <vilib>:"WPI_UltrasonicRefNum Registry Set.vi"("error in (no error)"=w18, "refnum name"=w16, "SonarMB1010AnalogDevRef"=w17) -> ()  [unwired: 7 in, 2 out]
